vi "Analyze Data.vi"   [LabVIEW 2018, in "RT - Analysis.lvlib"]
doc: "Runs all analysys on raw data to get calibrated and calculated values"
uses:
  RT - Analysis.lvlib
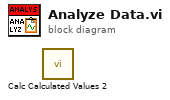
[diagram p0: block diagram]
diagram:
  n1 = call "Calc Calculated Values 2.vi"() -> ()  [unwired: 10 in, 2 out]
